vi "SupplySecurityWithoutP2X.vi"(8 "error in (no error)":errorcluster, 11 "DataFlowIN":T2) -> (0 "error out":errorcluster, 3 "DataFlowOUT":T2)   [LabVIEW 2019]
doc: "Subpanel Plugin VI that displays a random value, multiplied by a user-specified value, in a waveform chart."
uses:
  classes/DataCollector.lvclass
  classes/DataHandler.lvclass
panel:
  in  "Abfragegeschwindigkeit DB [ms]":i32=100
  out "Unload Limit":dbl
  out "Load Limit":dbl
  out "Bin-No.":u32
  out "Car enable Signal 2":bool
  out "Distance":bool
  out "E-Car":i32
  out "Car enable":bool
  out "Daytime":i32
  out "buffer":bool
  out "error out 2":errorcluster
  in  "Stopp":bool
  out "Car enable Signal":bool
  in  "Controlling":T1={"Prioritization"=0, "Operating Mode"="", "Release Time "={"Start"=0.0, "Stop"=0.0}, "Activity"=TRUE, " Limitation"={"CPC Power"=0.0, "Unload Power"=0.0, "Load Power"=0.0}}
  in  "Field Elements":i32(listbox)
  out "Control-Matrix-Overview":i32(listbox)=-1
  # "Zone 1 = Bin 1"
  # "Zone 2 = Bin 2"
  # "Zone 3 = Bin 4"
  # "DataCollector.lvclass:SelectValueDC.vi:Step on \"SELECT COUNT(*) FROM ThSorage\"\n\nSQLITE_BUSY(5): database is locked\n\nComplete Call Chain:\nDataCollector.lvclass:SelectValueDC.vi\nForecastNightDay.vi\nForecastSummerWinter.vi\nPrimaryEnergyMinimizationWithoutP2X.vi"
  # "DataCollector.lvclass:SelectValueDC.vi:Step on \"SELECT COUNT(*) FROM 'ElSorage_eCar'\"\n\nSQLITE_BUSY(5): database is locked\n\nComplete Call Chain:\nDataCollector.lvclass:SelectValueDC.vi\nPrimaryEnergyMinimizationWithoutP2X.vi"
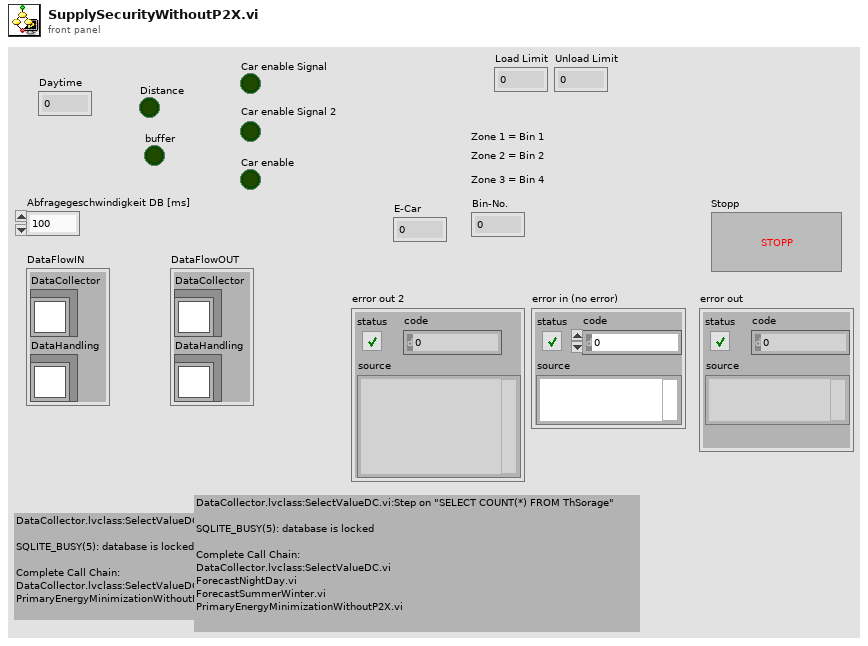
[diagram p1: front panel]
types:
  T1 = cluster{"Prioritization":i8, "Operating Mode":string, "Release Time ":cluster{"Start":dbl, "Stop":dbl}, "Activity":bool, " Limitation":cluster{"CPC Power":dbl, "Unload Power":dbl, "Load Power":dbl}}
  T2 = cluster{"DataCollector":refnum<class "DataCollector.lvclass">, "DataHandling":refnum<class "DataHandler.lvclass">}
  T3 = cluster{"Zone 1":cluster{"TOP_enable_Z1":dbl, "LOW_enable_Z1":dbl, "TOP_disable_Z1":dbl, "LOW_disable_Z1":dbl, "TOP_enable_crit__Z1":dbl, "LOW_enable_crit_Z1":dbl}, "Zone 2":cluster{"TOP_enable_Z2":dbl, "LOW_enable_Z2":dbl, "TOP_disable_Z2":dbl, "LOW_disable_Z2":dbl, "TOP_enable_crit__Z2":dbl, "LOW_enable_crit_Z2":dbl}, "Zone 3":cluster{"TOP_enable_Z3":dbl, "LOW_enable_Z3":dbl, "TOP_disable_Z3":dbl, "LOW_disable_Z3":dbl, "TOP_enable_crit__Z3":dbl, "LOW_enable_crit_Z3":dbl}}
  T4 = cluster{"Activity (on / off)":i64, "Prioritization":i64, "CPC Power Limit":dbl, "Unload Power Limit":dbl, "Load Power Limit":dbl, "Release Time":string, "Operating Mode":string}
  T5 = cluster{"DataCollector out":refnum<class "DataCollector.lvclass">, "DataHandler out":refnum<class "DataHandler.lvclass">}
  T6 = cluster{"TOP_enable_Z1":dbl, "LOW_enable_Z1":dbl, "TOP_disable_Z1":dbl, "LOW_disable_Z1":dbl, "TOP_enable_crit__Z1":dbl, "LOW_enable_crit_Z1":dbl}
  T7 = cluster{"TOP_enable_Z2":dbl, "LOW_enable_Z2":dbl, "TOP_disable_Z2":dbl, "LOW_disable_Z2":dbl, "TOP_enable_crit__Z2":dbl, "LOW_enable_crit_Z2":dbl}
  T8 = cluster{"TOP_enable_Z3":dbl, "LOW_enable_Z3":dbl, "TOP_disable_Z3":dbl, "LOW_disable_Z3":dbl, "TOP_enable_crit__Z3":dbl, "LOW_enable_crit_Z3":dbl}
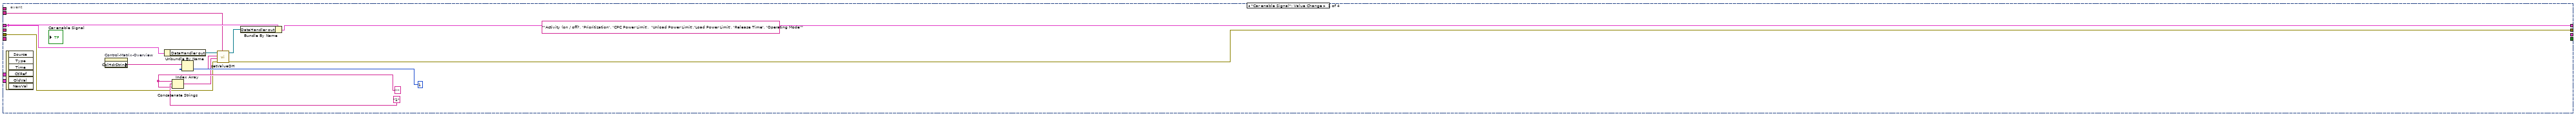
[diagram p2: hidden frame]
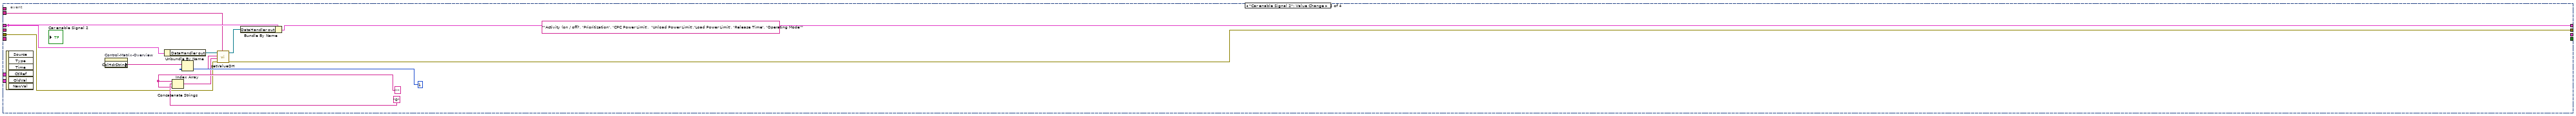
[diagram p3: hidden frame]
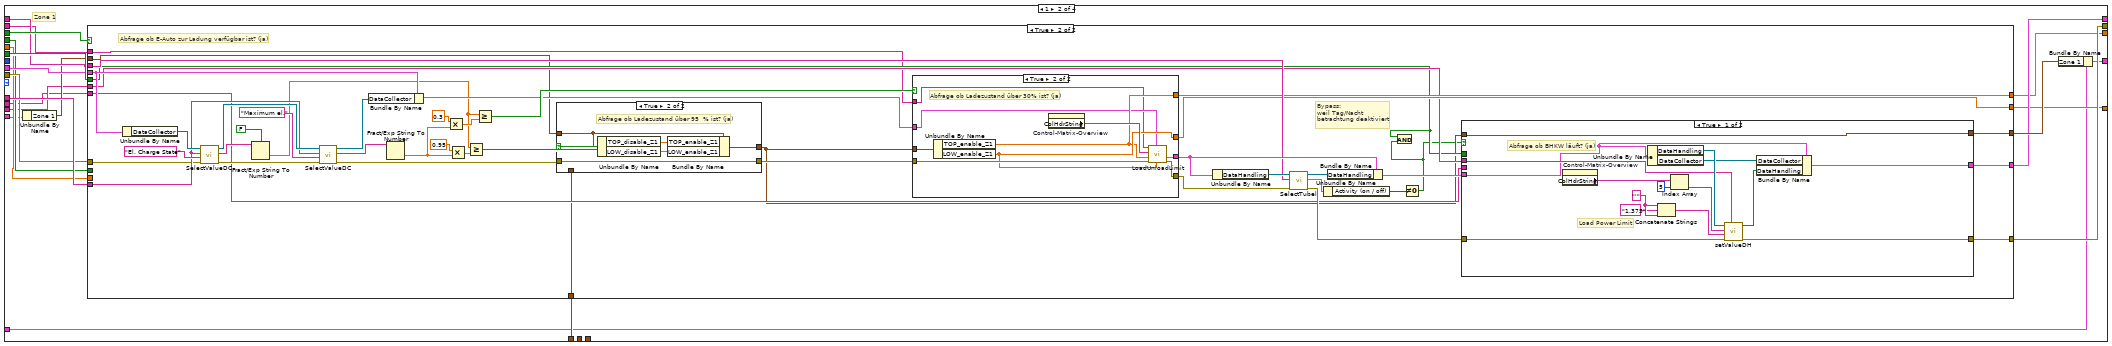
[diagram p5: hidden frame]
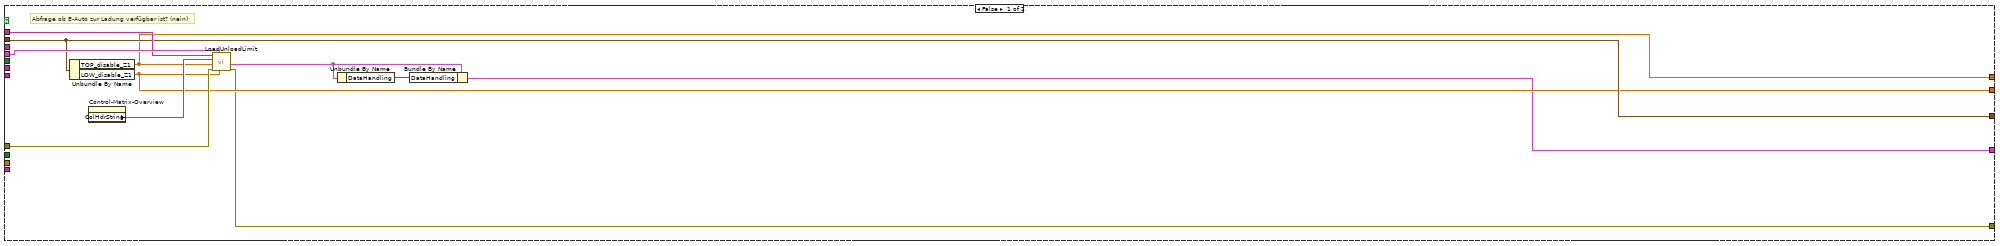
[diagram p6: hidden frame]
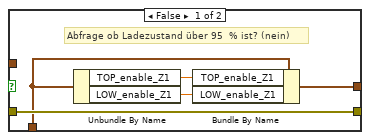
[diagram p7: hidden frame]
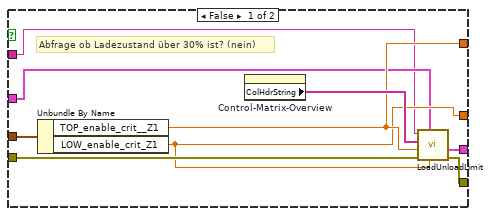
[diagram p8: hidden frame]
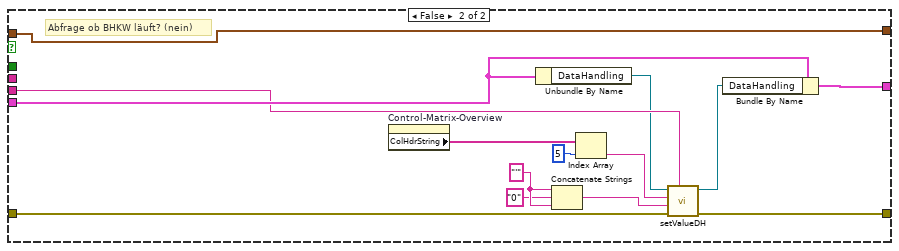
[diagram p9: hidden frame]
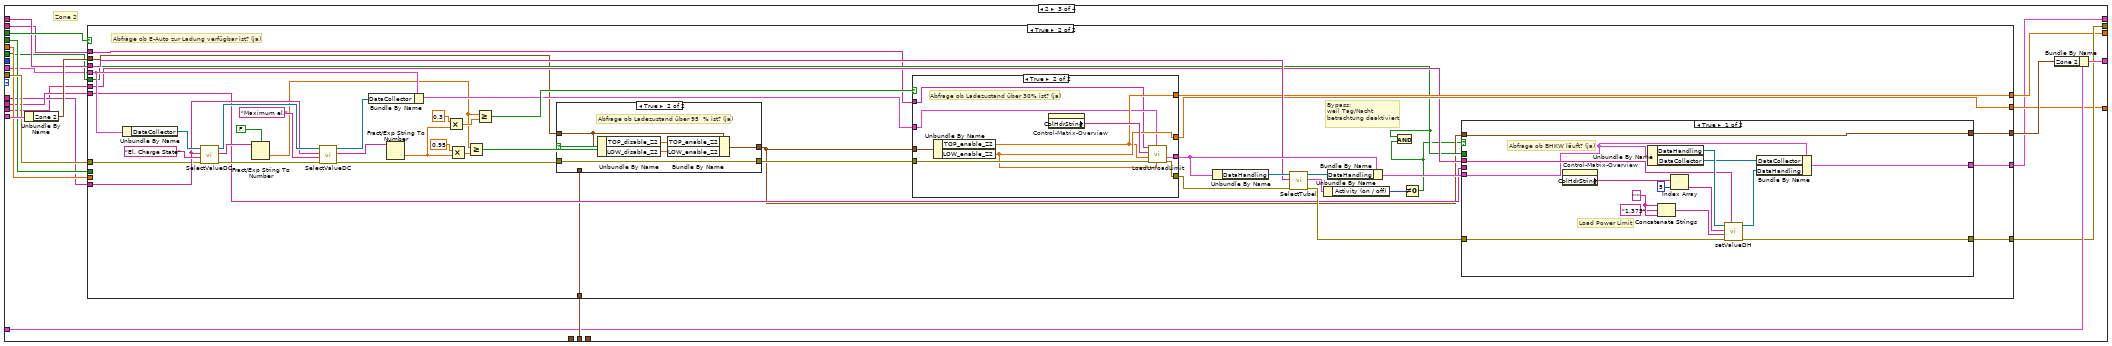
[diagram p10: hidden frame]
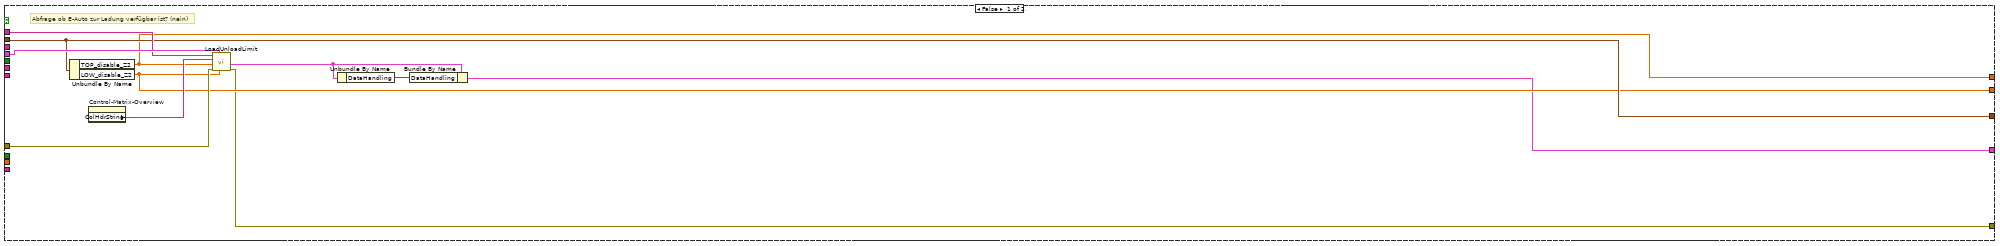
[diagram p11: hidden frame]
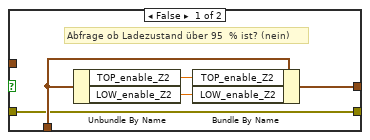
[diagram p12: hidden frame]
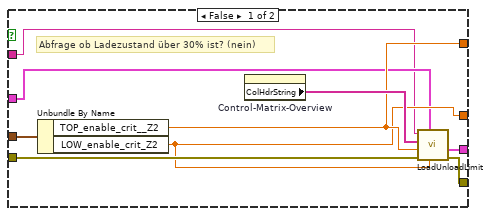
[diagram p13: hidden frame]
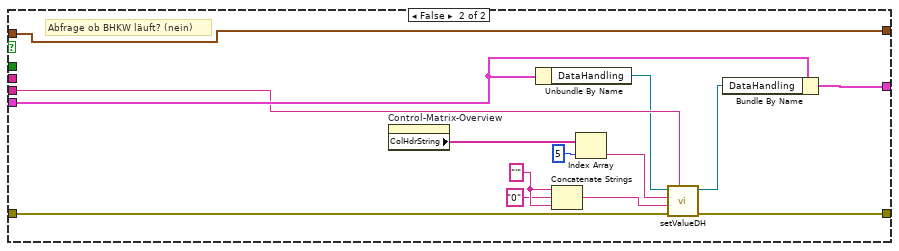
[diagram p14: hidden frame]
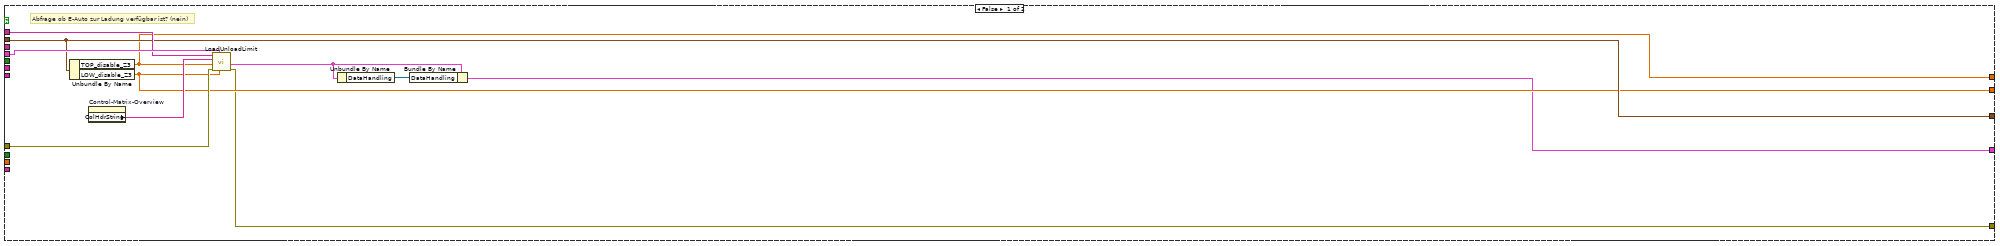
[diagram p15: hidden frame]
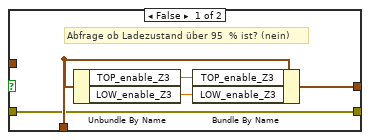
[diagram p16: hidden frame]
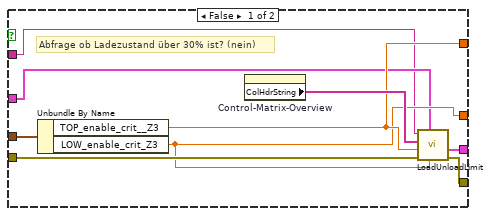
[diagram p17: hidden frame]
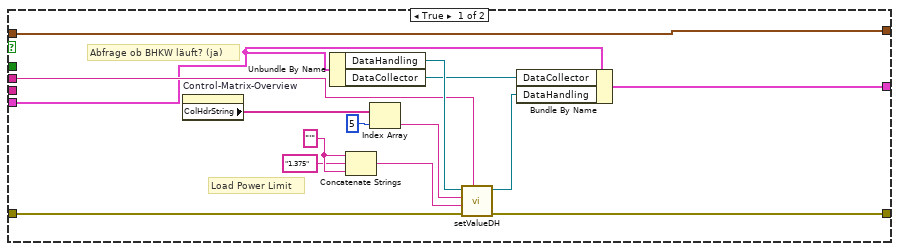
[diagram p18: hidden frame]
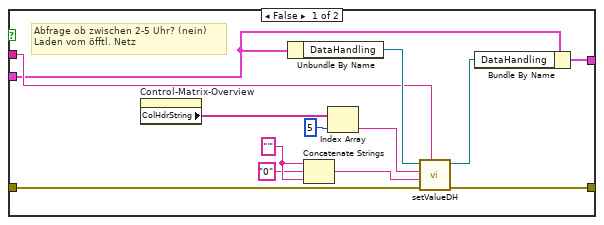
[diagram p19: hidden frame]
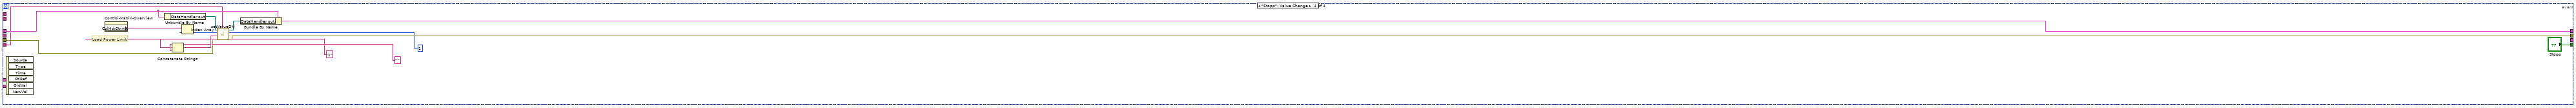
[diagram p20: hidden frame]
diagram:
  w5 = T3 {"Zone 1"={"TOP_enable_Z1"=55.0, "LOW_enable_Z1"=40.0, "TOP_disable_Z1"=50.0, "LOW_disable_Z1"=30.0, "TOP_enable_crit__Z1"=55.0, "LOW_enable_crit_Z1"=50.0}, "Zone 2"={"TOP_enable_Z2"=45.0, "LOW_enable_Z2"=40.0, "TOP_disable_Z2"=40.0, "LOW_disable_Z2"=30.0, "TOP_enable_crit__Z2"=50.0, "LOW_enable_crit_Z2"=45.0}, "Zone 3"={"TOP_enable_Z3"=40.0, "LOW_enable_Z3"=35.0, "TOP_disable_Z3"=35.0, "LOW_disable_Z3"=30.0, "TOP_enable_crit__Z3"=40.0, "LOW_enable_crit_Z3"=37.0}}
  w11 = TRUE
  (unwired) "'Daytime', 'Day of Year', 'El. Energy In',  'El. Energy Out', 'Th. Energy In',  'Th. Energy Out', 'Ch. Energy In',  'Ch. Energy Out',  'Maximum el.', 'Minimal el.', 'Maximum th.', 'Minimal th.',  'Maximum ch.', 'Minimal ch.', 'El. Capacity',  'Th. Capacity', 'Ch. Capacity', 'El. Charge State', 'Th. Charge State',  'Ch. Charge State', 'Activity (on / off)', 'Prioritization', 'El. Power Limitation',  'Th. Power Limitation', 'Ch. Power Limitation', 'Release Time', 'Operating Mode', 'e-Car Load Enable', 'e-Car Mileage  [km]'" ("string")
  w6 = "'CHP'" ("TableName")
  # "SQLite.lvlib:Connection.lvclass:Prepare (pointers).vi\nMAIN db name-->\"C:\\Users\\a_asfe0001\\Desktop\\CHPMobilityEnergySystem\\datebases\\e-car-management_controlling2.db\"\n\nSQLITE_ERROR(1): near \"618182\": syntax error\n\nComplete Call Chain:\nSQLite.lvlib:Connection.lvclass:Prepare (pointers).vi\nSQLite.lvlib:Connection.lvclass:Execute SQL (No results).vi:3980001\nDataHandler.lvclass:setValueDH.vi\nPrimaryEnergyMinimizationWithoutP2X.vi\n\nSQL: \"UPDATE ThSorage SET 'Load Power Limit' = 224,618182;\""
  n1 = case shown="True" w11 {
    tunnel: [w16 w34] -> w4
    tunnel: "error in (no error)" -> [w21 w33]
    tunnel: [w20 w27] -> w9
    tunnel: w6 -> [w19 w25]
    tunnel: [w17 w30] -> _
    frame False {
      n2 = Unbundle By Name("DataFlowIN") -> ("DataHandling"=w23:refnum<class "DataHandler.lvclass">)
      n3 = call-dynamic "SelectTubel.vi"("error in (no error)"=w21, "Unique Object Identifier"=w19, "DataHandler in"=w23) -> ("error out"=w20:errorcluster, "Control Parameter"=w24:T4, "DataHandler out"=w18:refnum<class "DataHandler.lvclass">)  [unwired: 5 in, 1 out]
      n4 = Unbundle By Name(w24) -> ("Activity (on / off)"=w17:i64)
      n5 = Bundle By Name(cluster="DataFlowIN", "DataHandling"=w18) -> (w16:T2)
    }
    frame True {
      w36 = refnum<class "DataHandler.lvclass"> refnum  # DataHandler.lvclass
      w41 = refnum<class "DataCollector.lvclass"> refnum  # DataCollector.lvclass
      n6 = call <vilib>:"Application Directory.vi"() -> ("Application Directory"=w44:path)
      n7 = Build Path(base path=w44, name or relative path="datebases\\e-car-management_monitoring_M12_SLP_gas_20000kWh_15min_500ms.db" ("Name oder relativer Pfad")) -> (appended path=w40:path)
      n8 = call <vilib>:"Application Directory.vi"() -> ("Application Directory"=w38:path)
      n9 = Build Path(base path=w38, name or relative path="datebases/e-car-management_controlling2.db" ("Name oder relativer Pfad")) -> (appended path=w35:path)
      n10 = call-dynamic "OpenCollector.vi"("error in (no error)"=w33, "Ram?"=FALSE, "path to db monitoring"=w40, "DataCollector in"=w41) -> ("error out"=w32:errorcluster, "DataCollector out"=w39:refnum<class "DataCollector.lvclass">)  [unwired: 5 in, 1 out]
      n11 = call-dynamic "OpenHandler.vi"("error in (no error)"=w32, "path to db monitoring"=w35, "DataHandling in"=w36) -> ("error out"=w26:errorcluster, "DataHandling out"=w28:refnum<class "DataHandler.lvclass">)  [unwired: 7 in]
      n12 = call-dynamic "SelectTubel.vi"("error in (no error)"=w26, "Unique Object Identifier"=w25, "DataHandler in"=w28) -> ("error out"=w27:errorcluster, "Control Parameter"=w31:T4, "DataHandler out"=w29:refnum<class "DataHandler.lvclass">)  [unwired: 5 in, 1 out]
      n13 = Unbundle By Name(w31) -> ("Activity (on / off)"=w30:i64)
      n14 = Bundle("DataCollector out"=w39, "DataHandler out"=w29) -> (w34:T5)  [unwired: 1 in]
    }
  }
  n15 = disable-structure shown="Aktiviert" {
    frame Disabled {
      n16 = property on="Eigenschaftsknoten" class="MehrSpaltFeld (strikt)"() -> ("ColHdrString"=w59:string[])  [unwired: 2 in, 2 out]
      n17 = Index Array(array=w59, index=2) -> (element=w57:string)
      n18 = Number To Decimal String(number=9 ("Zahl")) -> (decimal integer string=w60:string)  [unwired: 1 in]
      n19 = call "RestOperatingHoursEl.vi"() -> ("Fehler (Ausgang)"=w47:errorcluster, "DataFlowIN (Ausgang)"=w48:T2, "DataFlowIN (Eingang)"=w49:T2, "TableName"=w46:string)  [unwired: 7 in, 1 out]
      n20 = call-dynamic "setValueDH.vi"("error in (no error)"=w50, "Value"=w60, "ItemName"=w57, "DataHandler in"=w53) -> ("error out"=w55:errorcluster, "DataHandler out"=w52:refnum<class "DataHandler.lvclass">, "TableName"=w51:string)  [unwired: 5 in]
      n21 = call "RestOperatingHours.vi"("Fehler (Eingang, kein Fehler)"=w47, "DataFlowIN (Eingang)"=w48, "TableName"=w51) -> ("Fehler (Ausgang)"=w50:errorcluster, "DataFlowIN (Ausgang)"=w45:T2)  [unwired: 6 in, 1 out]
      n22 = Unbundle By Name(w45) -> ("DataHandling"=w53:refnum<class "DataHandler.lvclass">)
      n23 = Bundle By Name(cluster=w45, "DataHandling"=w52) -> (w54:T2)
    }
    frame Enabled {
    }
  }
  n24 = Unbundle By Name(w5) -> ("Zone 1"=w1:T6, "Zone 2"=w2:T7, "Zone 3"=w3:T8)
  n25 = while {
    tunnel: "ThSorage" ("TableName") -> [w77]
    tunnel: w6 -> [w76]
    tunnel: "'ElSorage_eCar'" ("TableName") -> [w64]
    tunnel: "'Consumer_EF'" ("TableName") -> [w75]
    shift-right: [w67] -> w8
    shift-left: w9 -> [w74]
    shift-right: [w72] -> w12
    shift-left: w4 -> [w71]
    shift-right: [w65] -> _
    shift-left: w5 -> [w66]
    tunnel: w3 -> [w63]
    tunnel: w2 -> [w62]
    tunnel: w1 -> [w61]
    stop <- w68 stop-if-true
    n26 = event shown="[2] Timeout" {
      selector: _ -> [_ _ _ _]
      dyn-events: _ -> [_ _ _ _]
      timeout: "Abfragegeschwindigkeit DB [ms]" -> [_ _ _ _]
      tunnel: w77 -> [_ _ w123 _]
      tunnel: [w90 w103 w110 w578] -> w67
      tunnel: w76 -> [w78 w91 w118 _]
      tunnel: w64 -> [_ _ w108 w575]
      tunnel: w75 -> [_ _ _ _]
      tunnel: w71 -> [w81 w94 w111 w577]
      tunnel: w74 -> [w80 w93 w138 w579]
      tunnel: [w89 w102 w148 w576] -> w72
      tunnel: [_ _ _ "Stopp"] -> w70
      tunnel: w66 -> [_ _ w114 _]
      tunnel: w66 -> [_ _ w113 _]
      tunnel: [_ _ w112 _] -> w65
      tunnel: w63 -> [_ _ w107 _]
      tunnel: w62 -> [_ _ w105 _]
      tunnel: w61 -> [_ _ w104 _]
      event "Car enable Signal": Value Change {
        w84 = "'" ("String")
        (unwired) "'Activity (on / off)', 'Prioritization', 'CPC Power Limit',  'Unload Power Limit','Load Power Limit', 'Release Time', 'Operating Mode'" ("string")
        n27 = event-data() -> ()  [unwired: 1 in, 6 out]
        n28 = property on="Control-Matrix-Overview" class="MehrSpaltFeld (strikt)"() -> ("ColHdrString"=w85:string[])  [unwired: 2 in, 2 out]
        n29 = Unbundle By Name(w81) -> ("DataHandler out"=w79:refnum<class "DataHandler.lvclass">)
        n30 = Concatenate Strings(w84, "1" ("String"), w84) -> (w83:string)
        n31 = Index Array(array=w85, index=1) -> (element=w87:string)
        n32 = call-dynamic "setValueDH.vi"("TableName"=w78, "error in (no error)"=w80, "Value"=w83, "ItemName"=w87, "DataHandler in"=w79) -> ("error out"=w90:errorcluster, "DataHandler out"=w86:refnum<class "DataHandler.lvclass">)  [unwired: 5 in]
        n33 = Bundle By Name(cluster=w81, "DataHandler out"=w86) -> (w89:T5)
      }
      event "Car enable Signal 2": Value Change {
        w97 = "'" ("String")
        (unwired) "'Activity (on / off)', 'Prioritization', 'CPC Power Limit',  'Unload Power Limit','Load Power Limit', 'Release Time', 'Operating Mode'" ("string")
        n34 = event-data() -> ()  [unwired: 1 in, 6 out]
        n35 = property on="Control-Matrix-Overview" class="MehrSpaltFeld (strikt)"() -> ("ColHdrString"=w98:string[])  [unwired: 2 in, 2 out]
        n36 = Unbundle By Name(w94) -> ("DataHandler out"=w92:refnum<class "DataHandler.lvclass">)
        n37 = Concatenate Strings(w97, "0" ("String"), w97) -> (w96:string)
        n38 = Index Array(array=w98, index=1) -> (element=w100:string)
        n39 = call-dynamic "setValueDH.vi"("TableName"=w91, "error in (no error)"=w93, "Value"=w96, "ItemName"=w100, "DataHandler in"=w92) -> ("error out"=w103:errorcluster, "DataHandler out"=w99:refnum<class "DataHandler.lvclass">)  [unwired: 5 in]
        n40 = Bundle By Name(cluster=w94, "DataHandler out"=w99) -> (w102:T5)
      }
      event Timeout {
        # "th"
        n41 = event-data() -> ()  [unwired: 1 in, 3 out]
        n42 = Unbundle By Name(w111) -> ("DataCollector out"=w144:refnum<class "DataCollector.lvclass">, "DataHandler out"=w140:refnum<class "DataHandler.lvclass">)
        n43 = call-dynamic "getControlMatrixDH.vi"("error in (no error)"=w138, "DataHandler in"=w140) -> ("error out"=w137:errorcluster, "List of ColHads"=w141:string[], "ControlParameterArrayMatrix"=w143:string[][], "DataHandler out"=w139:refnum<class "DataHandler.lvclass">, "Field Elements"=w142:string[])  [unwired: 5 in]
        n44 = property on="Field Elements" class="Listenfeld (strikt)"("Item Names"=w142) -> ()  [unwired: 2 in, 2 out]
        n45 = property on="Control-Matrix-Overview" class="MehrSpaltFeld (strikt)"("ItemNames"=w143) -> ()  [unwired: 2 in, 2 out]
        n46 = property on="Control-Matrix-Overview" class="MehrSpaltFeld (strikt)"("ColHdrString"=w141) -> ()  [unwired: 2 in, 2 out]
        n47 = call-dynamic "SelectValueDC.vi"("error in (no error)"=w137, "Table Row Name"="e-Car Load Enable", "Unique Object Identifier"=w108, "DataCollector in"=w144) -> ("error out"=w134:errorcluster, "Value"=w145:string, "DataCollector out"=w135:refnum<class "DataCollector.lvclass">)  [unwired: 5 in]
        n48 = call-dynamic "SelectValueDC.vi"("error in (no error)"=w134, "Table Row Name"="e-Car Mileage  [km]", "Unique Object Identifier"=w108, "DataCollector in"=w135) -> ("error out"=w126:errorcluster, "Value"=w133:string, "DataCollector out"=w128:refnum<class "DataCollector.lvclass">)  [unwired: 5 in]
        n49 = Decimal String To Number(string=w145) -> (number=w146:i32)  [unwired: 2 in, 1 out]
        "E-Car" <- w146
        n50 = Decimal String To Number(string=w133) -> (number=w132:i32)  [unwired: 2 in, 1 out]
        n51 = call-dynamic "SelectValueDC.vi"("error in (no error)"=w126, "Table Row Name"="Th. Charge State", "Unique Object Identifier"=w123, "DataCollector in"=w128) -> ("error out"=w122:errorcluster, "Value"=w106:string, "DataCollector out"=w127:refnum<class "DataCollector.lvclass">)  [unwired: 5 in]
        n52 = Bundle By Name(cluster=w111, "DataCollector out"=w127, "DataHandler out"=w139) -> (w121:T5)
        n53 = Fract/Exp String To Number(string=w106) -> (number=w129:dbl)  [unwired: 3 in, 1 out]
        n54 = Not Equal To 0?(x=w146) -> (x != 0?=w136:bool)
        "Car enable" <- w136
        n55 = Not Equal To 0?(x=w132) -> (x != 0?=w109:bool)
        "Distance" <- w109
        n56 = call "ForecastSummerWinter.vi"("Fehler (Eingang, kein Fehler)"=w122, "DataFlowIN (Eingang)"=w121, "TableName"=w123) -> ("Fehler (Ausgang)"=w124:errorcluster, "DataFlowIN (Ausgang)"=w125:T2, "Daytime"=w120:i32, "Bin-No."=w119:u32, "Night(22-6)?"=w115:bool)  [unwired: 1 in, 3 out]
        "Daytime" <- w120
        "Bin-No." <- w119
        n57 = case shown="4" w119 {
          tunnel: [w151 w157 w286 w428] -> w148
          tunnel: w136 -> [_ w172 w306 w437]
          tunnel: w108 -> [_ w161 w295 w431]
          tunnel: w109 -> [_ w165 w301 w436]
          tunnel: w129 -> [_ w164 w300 w435]
          tunnel: w125 -> [w151 w167 w298 w430]
          tunnel: w124 -> [w150 w166 w303 w438]
          tunnel: w123 -> [_ w168 w294 w433]
          tunnel: w120 -> [_ _ _ _]
          tunnel: w115 -> [_ w171 w299 w429]
          tunnel: w118 -> [_ w169 w302 w434]
          tunnel: [_ w154 w287 w420] -> w117
          tunnel: [_ w155 w288 w427] -> w116
          tunnel: w108 -> [_ w160 w297 w432]
          tunnel: w114 -> [_ w163 w305 w440]
          tunnel: w113 -> [w149 w152 w290 w425]
          tunnel: [w149 w153 w292 w424] -> w112
          tunnel: [w150 w156 w289 w421] -> w110
          tunnel: w108 -> [_ w170 w296 w423]
          tunnel: w107 -> [_ _ _ w422]
          tunnel: w105 -> [_ _ w291 _]
          tunnel: w104 -> [_ w159 _ _]
          frame 0, Default {
          }
          frame 1 {
            # "Zone 1"
            n58 = Unbundle By Name(w163) -> ("Zone 1"=w162:T6)
            n59 = case shown="True" w172 {
              tunnel: [w174 w227] -> w157
              tunnel: [w173 w228] -> w156
              tunnel: w161 -> [_ w197]
              tunnel: w166 -> [w182 w204]
              tunnel: w167 -> [w181 w203]
              tunnel: w168 -> [w179 w186]
              tunnel: w171 -> [_ w196]
              tunnel: w169 -> [_ w206]
              tunnel: [w176 w202] -> w155
              tunnel: w160 -> [_ w198]
              tunnel: w162 -> [w177 w188]
              tunnel: [w177 w226] -> w158
              tunnel: w170 -> [_ w205]
              tunnel: w165 -> [_ _]
              tunnel: w164 -> [_ _]
              tunnel: w159 -> [_ w184]
              tunnel: [w175 w201] -> w154
              frame False {
                # "Abfrage ob E-Auto zur Ladung verfügbar ist? (nein)"
                n60 = Unbundle By Name(w177) -> ("TOP_disable_Z1"=w175:dbl, "LOW_disable_Z1"=w176:dbl)
                n61 = property on="Control-Matrix-Overview" class="MehrSpaltFeld (strikt)"() -> ("ColHdrString"=w178:string[])  [unwired: 2 in, 2 out]
                n62 = call "LoadUnloadLimit.vi"("Unload Limit"=w176, "DataFlowIN (Eingang)"=w181, "Fehler (Eingang, kein Fehler)"=w182, "Load Limit"=w175, "ColHdrString"=w178, "TableName"=w179) -> ("Fehler (Ausgang)"=w173:errorcluster, "DataFlowIN (Ausgang)"=w180:T2)  [unwired: 2 in, 2 out]
                n63 = Unbundle By Name(w180) -> ("DataHandling"=w183:refnum<class "DataHandler.lvclass">)
                n64 = Bundle By Name(cluster=w180, "DataHandling"=w183) -> (w174:T2)
              }
              frame True {
                # "Bypass:\nweil Tag/Nacht \nbetrachtung deaktiviert"
                # "Abfrage ob E-Auto zur Ladung verfügbar ist? (ja)"
                n65 = Unbundle By Name(w203) -> ("DataCollector"=w216:refnum<class "DataCollector.lvclass">)
                n66 = call-dynamic "SelectValueDC.vi"("error in (no error)"=w204, "Table Row Name"="El. Charge State", "Unique Object Identifier"=w205, "DataCollector in"=w216) -> ("error out"=w212:errorcluster, "Value"=w213:string, "DataCollector out"=w215:refnum<class "DataCollector.lvclass">)  [unwired: 5 in]
                n67 = Fract/Exp String To Number(use system decimal point (T)=FALSE ("Systemdezimalzeichen verwenden (T)"), string=w213) -> (number=w192:dbl)  [unwired: 2 in, 1 out]
                n68 = call-dynamic "SelectValueDC.vi"("error in (no error)"=w212, "Table Row Name"="Maximum el.", "Unique Object Identifier"=w205, "DataCollector in"=w215) -> ("error out"=w190:errorcluster, "Value"=w211:string, "DataCollector out"=w214:refnum<class "DataCollector.lvclass">)  [unwired: 5 in]
                n69 = Bundle By Name(cluster=w203, "DataCollector"=w214) -> (w217:T2)
                n70 = Fract/Exp String To Number(string=w211) -> (number=w193:dbl)  [unwired: 3 in, 1 out]
                n71 = Multiply(x=0.3 ("x*y"), y=w193) -> (x*y=w219:dbl)
                n72 = Multiply(x=0.95 ("x*y"), y=w193) -> (x*y=w194:dbl)
                n73 = Greater Or Equal?(x=w192, y=w194) -> (x >= y?=w191:bool)
                n74 = Greater Or Equal?(x=w192, y=w219) -> (x >= y?=w218:bool)
                n75 = case shown="True" w191 {
                  tunnel: w188 -> [_ w234]
                  tunnel: [w231 w235] -> w187
                  tunnel: [w230 w238] -> w189
                  tunnel: w190 -> [w230 w238]
                  tunnel: w184 -> [w229 _]
                  frame False {
                    # "Abfrage ob Ladezustand über 95  % ist? (nein)"
                    n76 = Unbundle By Name(w229) -> ("TOP_enable_Z1"=w232:dbl, "LOW_enable_Z1"=w233:dbl)
                    n77 = Bundle By Name(cluster=w229, "TOP_enable_Z1"=w232, "LOW_enable_Z1"=w233) -> (w231:T6)
                  }
                  frame True {
                    # "Abfrage ob Ladezustand über 95  % ist? (ja)"
                    n78 = Unbundle By Name(w234) -> ("TOP_disable_Z1"=w236:dbl, "LOW_disable_Z1"=w237:dbl)
                    n79 = Bundle By Name(cluster=w234, "TOP_enable_Z1"=w236, "LOW_enable_Z1"=w237) -> (w235:T6)
                  }
                }
                n80 = case shown="True" w218 {
                  tunnel: [w243 w251] -> w221
                  tunnel: w217 -> [w240 w250]
                  tunnel: w189 -> [w246 w255]
                  tunnel: [w242 w252] -> w220
                  tunnel: [w245 w253] -> w201
                  tunnel: [w244 w254] -> w202
                  tunnel: w186 -> [w239 w249]
                  tunnel: w187 -> [w241 w248]
                  frame False {
                    # "Abfrage ob Ladezustand über 30% ist? (nein)"
                    n81 = Unbundle By Name(w241) -> ("TOP_enable_crit__Z1"=w245:dbl, "LOW_enable_crit_Z1"=w244:dbl)
                    n82 = property on="Control-Matrix-Overview" class="MehrSpaltFeld (strikt)"() -> ("ColHdrString"=w247:string[])  [unwired: 2 in, 2 out]
                    n83 = call "LoadUnloadLimit.vi"("Unload Limit"=w244, "DataFlowIN (Eingang)"=w240, "Fehler (Eingang, kein Fehler)"=w246, "Load Limit"=w245, "ColHdrString"=w247, "TableName"=w239) -> ("Fehler (Ausgang)"=w242:errorcluster, "DataFlowIN (Ausgang)"=w243:T2)  [unwired: 2 in, 2 out]
                  }
                  frame True {
                    # "Abfrage ob Ladezustand über 30% ist? (ja)"
                    n84 = Unbundle By Name(w248) -> ("TOP_enable_Z1"=w253:dbl, "LOW_enable_Z1"=w254:dbl)
                    n85 = property on="Control-Matrix-Overview" class="MehrSpaltFeld (strikt)"() -> ("ColHdrString"=w256:string[])  [unwired: 2 in, 2 out]
                    n86 = call "LoadUnloadLimit.vi"("Unload Limit"=w254, "DataFlowIN (Eingang)"=w250, "Fehler (Eingang, kein Fehler)"=w255, "Load Limit"=w253, "ColHdrString"=w256, "TableName"=w249) -> ("Fehler (Ausgang)"=w252:errorcluster, "DataFlowIN (Ausgang)"=w251:T2)  [unwired: 2 in, 2 out]
                  }
                }
                n87 = Unbundle By Name(w221) -> ("DataHandling"=w225:refnum<class "DataHandler.lvclass">)
                n88 = call-dynamic "SelectTubel.vi"("error in (no error)"=w220, "Unique Object Identifier"=w206, "DataHandler in"=w225) -> ("error out"=w200:errorcluster, "Control Parameter"=w223:T4, "DataHandler out"=w224:refnum<class "DataHandler.lvclass">)  [unwired: 5 in, 1 out]
                n89 = Unbundle By Name(w223) -> ("Activity (on / off)"=w222:i64)
                n90 = Bundle By Name(cluster=w221, "DataHandling"=w224) -> (w199:T2)
                n91 = Not Equal To 0?(x=w222) -> (x != 0?=w185:bool)
                n92 = And(x=w196, y=w185) -> ()  [unwired: 1 out]
                n93 = case shown="True" w185 {
                  tunnel: [w261 w285] -> w228
                  tunnel: [w257 w284] -> w227
                  tunnel: w197 -> [w267 _]
                  tunnel: w200 -> [w265 w283]
                  tunnel: w199 -> [w258 w282]
                  tunnel: w198 -> [_ w281]
                  tunnel: w187 -> [w262 w280]
                  tunnel: [w262 w280] -> w226
                  tunnel: w196 -> [_ _]
                  frame True {
                    w266 = "'" ("String")
                    # "Abfrage ob BHKW läuft? (ja)"
                    # "Load Power Limit"
                    n94 = property on="Control-Matrix-Overview" class="MehrSpaltFeld (strikt)"() -> ("ColHdrString"=w263:string[])  [unwired: 2 in, 2 out]
                    n95 = Unbundle By Name(w258) -> ("DataHandling"=w268:refnum<class "DataHandler.lvclass">, "DataCollector"=w260:refnum<class "DataCollector.lvclass">)
                    n96 = Concatenate Strings(w266, "1.375" ("String"), w266) -> (w269:string)
                    n97 = Index Array(array=w263, index=5) -> (element=w270:string)
                    n98 = call-dynamic "setValueDH.vi"("TableName"=w267, "error in (no error)"=w265, "Value"=w269, "ItemName"=w270, "DataHandler in"=w268) -> ("error out"=w261:errorcluster, "DataHandler out"=w259:refnum<class "DataHandler.lvclass">)  [unwired: 5 in]
                    n99 = Bundle By Name(cluster=w258, "DataCollector"=w260, "DataHandling"=w259) -> (w257:T2)
                  }
                  frame False {
                    w274 = "'" ("String")
                    # "Abfrage ob BHKW läuft? (nein)"
                    n100 = property on="Control-Matrix-Overview" class="MehrSpaltFeld (strikt)"() -> ("ColHdrString"=w272:string[])  [unwired: 2 in, 2 out]
                    n101 = Unbundle By Name(w282) -> ("DataHandling"=w279:refnum<class "DataHandler.lvclass">)
                    n102 = Concatenate Strings(w274, "0" ("String"), w274) -> (w276:string)
                    n103 = Index Array(array=w272, index=5) -> (element=w278:string)
                    n104 = call-dynamic "setValueDH.vi"("TableName"=w281, "error in (no error)"=w283, "Value"=w276, "ItemName"=w278, "DataHandler in"=w279) -> ("error out"=w285:errorcluster, "DataHandler out"=w277:refnum<class "DataHandler.lvclass">)  [unwired: 5 in]
                    n105 = Bundle By Name(cluster=w282, "DataHandling"=w277) -> (w284:T2)
                  }
                }
              }
            }
            n106 = Bundle By Name(cluster=w152, "Zone 1"=w158) -> (w153:T3)
          }
          frame 2 {
            # "Zone 2"
            n107 = Unbundle By Name(w305) -> ("Zone 2"=w304:T7)
            n108 = case shown="True" w306 {
              tunnel: [w308 w361] -> w286
              tunnel: [w307 w362] -> w289
              tunnel: w295 -> [_ w331]
              tunnel: w303 -> [w316 w338]
              tunnel: w298 -> [w315 w337]
              tunnel: w294 -> [w313 w320]
              tunnel: w299 -> [_ w330]
              tunnel: w302 -> [_ w340]
              tunnel: [w309 w335] -> w287
              tunnel: [w310 w336] -> w288
              tunnel: w297 -> [_ w332]
              tunnel: w304 -> [w311 w322]
              tunnel: [w311 w360] -> w293
              tunnel: w296 -> [_ w339]
              tunnel: w301 -> [_ _]
              tunnel: w300 -> [_ _]
              tunnel: w291 -> [_ w318]
              frame False {
                # "Abfrage ob E-Auto zur Ladung verfügbar ist? (nein)"
                n109 = Unbundle By Name(w311) -> ("TOP_disable_Z2"=w309:dbl, "LOW_disable_Z2"=w310:dbl)
                n110 = property on="Control-Matrix-Overview" class="MehrSpaltFeld (strikt)"() -> ("ColHdrString"=w312:string[])  [unwired: 2 in, 2 out]
                n111 = call "LoadUnloadLimit.vi"("Unload Limit"=w310, "DataFlowIN (Eingang)"=w315, "Fehler (Eingang, kein Fehler)"=w316, "Load Limit"=w309, "ColHdrString"=w312, "TableName"=w313) -> ("Fehler (Ausgang)"=w307:errorcluster, "DataFlowIN (Ausgang)"=w314:T2)  [unwired: 2 in, 2 out]
                n112 = Unbundle By Name(w314) -> ("DataHandling"=w317:refnum<class "DataHandler.lvclass">)
                n113 = Bundle By Name(cluster=w314, "DataHandling"=w317) -> (w308:T2)
              }
              frame True {
                # "Bypass:\nweil Tag/Nacht \nbetrachtung deaktiviert"
                # "Abfrage ob E-Auto zur Ladung verfügbar ist? (ja)"
                n114 = Unbundle By Name(w337) -> ("DataCollector"=w350:refnum<class "DataCollector.lvclass">)
                n115 = call-dynamic "SelectValueDC.vi"("error in (no error)"=w338, "Table Row Name"="El. Charge State", "Unique Object Identifier"=w339, "DataCollector in"=w350) -> ("error out"=w346:errorcluster, "Value"=w347:string, "DataCollector out"=w349:refnum<class "DataCollector.lvclass">)  [unwired: 5 in]
                n116 = Fract/Exp String To Number(use system decimal point (T)=FALSE ("Systemdezimalzeichen verwenden (T)"), string=w347) -> (number=w326:dbl)  [unwired: 2 in, 1 out]
                n117 = call-dynamic "SelectValueDC.vi"("error in (no error)"=w346, "Table Row Name"="Maximum el.", "Unique Object Identifier"=w339, "DataCollector in"=w349) -> ("error out"=w324:errorcluster, "Value"=w345:string, "DataCollector out"=w348:refnum<class "DataCollector.lvclass">)  [unwired: 5 in]
                n118 = Bundle By Name(cluster=w337, "DataCollector"=w348) -> (w351:T2)
                n119 = Fract/Exp String To Number(string=w345) -> (number=w327:dbl)  [unwired: 3 in, 1 out]
                n120 = Multiply(x=0.3 ("x*y"), y=w327) -> (x*y=w353:dbl)
                n121 = Multiply(x=0.95 ("x*y"), y=w327) -> (x*y=w328:dbl)
                n122 = Greater Or Equal?(x=w326, y=w328) -> (x >= y?=w325:bool)
                n123 = Greater Or Equal?(x=w326, y=w353) -> (x >= y?=w352:bool)
                n124 = case shown="True" w325 {
                  tunnel: w322 -> [_ w368]
                  tunnel: [w365 w369] -> w321
                  tunnel: w318 -> [w364 _]
                  tunnel: [w363 w372] -> w323
                  tunnel: w324 -> [w363 w372]
                  frame False {
                    # "Abfrage ob Ladezustand über 95  % ist? (nein)"
                    n125 = Unbundle By Name(w364) -> ("TOP_enable_Z2"=w366:dbl, "LOW_enable_Z2"=w367:dbl)
                    n126 = Bundle By Name(cluster=w364, "TOP_enable_Z2"=w366, "LOW_enable_Z2"=w367) -> (w365:T7)
                  }
                  frame True {
                    # "Abfrage ob Ladezustand über 95  % ist? (ja)"
                    n127 = Unbundle By Name(w368) -> ("TOP_disable_Z2"=w370:dbl, "LOW_disable_Z2"=w371:dbl)
                    n128 = Bundle By Name(cluster=w368, "TOP_enable_Z2"=w370, "LOW_enable_Z2"=w371) -> (w369:T7)
                  }
                }
                n129 = case shown="True" w352 {
                  tunnel: [w377 w385] -> w355
                  tunnel: w351 -> [w374 w384]
                  tunnel: w323 -> [w380 w389]
                  tunnel: [w376 w386] -> w354
                  tunnel: [w379 w387] -> w335
                  tunnel: [w378 w388] -> w336
                  tunnel: w320 -> [w373 w383]
                  tunnel: w321 -> [w375 w382]
                  frame False {
                    # "Abfrage ob Ladezustand über 30% ist? (nein)"
                    n130 = Unbundle By Name(w375) -> ("TOP_enable_crit__Z2"=w379:dbl, "LOW_enable_crit_Z2"=w378:dbl)
                    n131 = property on="Control-Matrix-Overview" class="MehrSpaltFeld (strikt)"() -> ("ColHdrString"=w381:string[])  [unwired: 2 in, 2 out]
                    n132 = call "LoadUnloadLimit.vi"("Unload Limit"=w378, "DataFlowIN (Eingang)"=w374, "Fehler (Eingang, kein Fehler)"=w380, "Load Limit"=w379, "ColHdrString"=w381, "TableName"=w373) -> ("Fehler (Ausgang)"=w376:errorcluster, "DataFlowIN (Ausgang)"=w377:T2)  [unwired: 2 in, 2 out]
                  }
                  frame True {
                    # "Abfrage ob Ladezustand über 30% ist? (ja)"
                    n133 = Unbundle By Name(w382) -> ("TOP_enable_Z2"=w387:dbl, "LOW_enable_Z2"=w388:dbl)
                    n134 = property on="Control-Matrix-Overview" class="MehrSpaltFeld (strikt)"() -> ("ColHdrString"=w390:string[])  [unwired: 2 in, 2 out]
                    n135 = call "LoadUnloadLimit.vi"("Unload Limit"=w388, "DataFlowIN (Eingang)"=w384, "Fehler (Eingang, kein Fehler)"=w389, "Load Limit"=w387, "ColHdrString"=w390, "TableName"=w383) -> ("Fehler (Ausgang)"=w386:errorcluster, "DataFlowIN (Ausgang)"=w385:T2)  [unwired: 2 in, 2 out]
                  }
                }
                n136 = Unbundle By Name(w355) -> ("DataHandling"=w359:refnum<class "DataHandler.lvclass">)
                n137 = call-dynamic "SelectTubel.vi"("error in (no error)"=w354, "Unique Object Identifier"=w340, "DataHandler in"=w359) -> ("error out"=w334:errorcluster, "Control Parameter"=w357:T4, "DataHandler out"=w358:refnum<class "DataHandler.lvclass">)  [unwired: 5 in, 1 out]
                n138 = Unbundle By Name(w357) -> ("Activity (on / off)"=w356:i64)
                n139 = Bundle By Name(cluster=w355, "DataHandling"=w358) -> (w333:T2)
                n140 = Not Equal To 0?(x=w356) -> (x != 0?=w319:bool)
                n141 = And(x=w330, y=w319) -> ()  [unwired: 1 out]
                n142 = case shown="True" w319 {
                  tunnel: [w395 w419] -> w362
                  tunnel: [w391 w418] -> w361
                  tunnel: w331 -> [w401 _]
                  tunnel: w334 -> [w399 w417]
                  tunnel: w333 -> [w392 w416]
                  tunnel: w332 -> [_ w415]
                  tunnel: w321 -> [w396 w414]
                  tunnel: [w396 w414] -> w360
                  tunnel: w330 -> [_ _]
                  frame True {
                    w400 = "'" ("String")
                    # "Abfrage ob BHKW läuft? (ja)"
                    # "Load Power Limit"
                    n143 = property on="Control-Matrix-Overview" class="MehrSpaltFeld (strikt)"() -> ("ColHdrString"=w397:string[])  [unwired: 2 in, 2 out]
                    n144 = Unbundle By Name(w392) -> ("DataHandling"=w402:refnum<class "DataHandler.lvclass">, "DataCollector"=w394:refnum<class "DataCollector.lvclass">)
                    n145 = Concatenate Strings(w400, "1.375" ("String"), w400) -> (w403:string)
                    n146 = Index Array(array=w397, index=5) -> (element=w404:string)
                    n147 = call-dynamic "setValueDH.vi"("TableName"=w401, "error in (no error)"=w399, "Value"=w403, "ItemName"=w404, "DataHandler in"=w402) -> ("error out"=w395:errorcluster, "DataHandler out"=w393:refnum<class "DataHandler.lvclass">)  [unwired: 5 in]
                    n148 = Bundle By Name(cluster=w392, "DataCollector"=w394, "DataHandling"=w393) -> (w391:T2)
                  }
                  frame False {
                    w408 = "'" ("String")
                    # "Abfrage ob BHKW läuft? (nein)"
                    n149 = property on="Control-Matrix-Overview" class="MehrSpaltFeld (strikt)"() -> ("ColHdrString"=w406:string[])  [unwired: 2 in, 2 out]
                    n150 = Unbundle By Name(w416) -> ("DataHandling"=w413:refnum<class "DataHandler.lvclass">)
                    n151 = Concatenate Strings(w408, "0" ("String"), w408) -> (w410:string)
                    n152 = Index Array(array=w406, index=5) -> (element=w412:string)
                    n153 = call-dynamic "setValueDH.vi"("TableName"=w415, "error in (no error)"=w417, "Value"=w410, "ItemName"=w412, "DataHandler in"=w413) -> ("error out"=w419:errorcluster, "DataHandler out"=w411:refnum<class "DataHandler.lvclass">)  [unwired: 5 in]
                    n154 = Bundle By Name(cluster=w416, "DataHandling"=w411) -> (w418:T2)
                  }
                }
              }
            }
            n155 = Bundle By Name(cluster=w290, "Zone 2"=w293) -> (w292:T3)
          }
          frame 4 {
            # "Zone 3"
            n156 = Unbundle By Name(w440) -> ("Zone 3"=w439:T8)
            n157 = case shown="True" w437 {
              tunnel: [w442 w495] -> w428
              tunnel: [w441 w496] -> w421
              tunnel: w431 -> [_ w465]
              tunnel: w438 -> [w450 w472]
              tunnel: w430 -> [w449 w471]
              tunnel: w433 -> [w447 w453]
              tunnel: w429 -> [_ w464]
              tunnel: w434 -> [_ w474]
              tunnel: [w443 w469] -> w420
              tunnel: [w444 w470] -> w427
              tunnel: w432 -> [_ w466]
              tunnel: w439 -> [w445 w455]
              tunnel: [w445 w494] -> w426
              tunnel: w436 -> [_ _]
              tunnel: w435 -> [_ _]
              tunnel: w423 -> [_ w473]
              tunnel: w422 -> [_ w458]
              frame False {
                # "Abfrage ob E-Auto zur Ladung verfügbar ist? (nein)"
                n158 = Unbundle By Name(w445) -> ("TOP_disable_Z3"=w443:dbl, "LOW_disable_Z3"=w444:dbl)
                n159 = property on="Control-Matrix-Overview" class="MehrSpaltFeld (strikt)"() -> ("ColHdrString"=w446:string[])  [unwired: 2 in, 2 out]
                n160 = call "LoadUnloadLimit.vi"("Unload Limit"=w444, "DataFlowIN (Eingang)"=w449, "Fehler (Eingang, kein Fehler)"=w450, "Load Limit"=w443, "ColHdrString"=w446, "TableName"=w447) -> ("Fehler (Ausgang)"=w441:errorcluster, "DataFlowIN (Ausgang)"=w448:T2)  [unwired: 2 in, 2 out]
                n161 = Unbundle By Name(w448) -> ("DataHandling"=w451:refnum<class "DataHandler.lvclass">)
                n162 = Bundle By Name(cluster=w448, "DataHandling"=w451) -> (w442:T2)
              }
              frame True {
                # "Bypass:\nweil Tag/Nacht \nbetrachtung deaktiviert"
                # "Abfrage ob E-Auto zur Ladung verfügbar ist? (ja)"
                n163 = Unbundle By Name(w471) -> ("DataCollector"=w484:refnum<class "DataCollector.lvclass">)
                n164 = call-dynamic "SelectValueDC.vi"("error in (no error)"=w472, "Table Row Name"="El. Charge State", "Unique Object Identifier"=w473, "DataCollector in"=w484) -> ("error out"=w480:errorcluster, "Value"=w481:string, "DataCollector out"=w483:refnum<class "DataCollector.lvclass">)  [unwired: 5 in]
                n165 = Fract/Exp String To Number(use system decimal point (T)=FALSE ("Systemdezimalzeichen verwenden (T)"), string=w481) -> (number=w460:dbl)  [unwired: 2 in, 1 out]
                n166 = call-dynamic "SelectValueDC.vi"("error in (no error)"=w480, "Table Row Name"="Maximum el.", "Unique Object Identifier"=w473, "DataCollector in"=w483) -> ("error out"=w457:errorcluster, "Value"=w479:string, "DataCollector out"=w482:refnum<class "DataCollector.lvclass">)  [unwired: 5 in]
                n167 = Bundle By Name(cluster=w471, "DataCollector"=w482) -> (w485:T2)
                n168 = Fract/Exp String To Number(string=w479) -> (number=w461:dbl)  [unwired: 3 in, 1 out]
                n169 = Multiply(x=0.3 ("x*y"), y=w461) -> (x*y=w487:dbl)
                n170 = Multiply(x=0.95 ("x*y"), y=w461) -> (x*y=w462:dbl)
                n171 = Greater Or Equal?(x=w460, y=w462) -> (x >= y?=w459:bool)
                n172 = Greater Or Equal?(x=w460, y=w487) -> (x >= y?=w486:bool)
                n173 = case shown="True" w459 {
                  tunnel: w455 -> [_ w502]
                  tunnel: [w499 w503] -> w454
                  tunnel: w458 -> [w498 _]
                  tunnel: [w497 w506] -> w456
                  tunnel: w457 -> [w497 w506]
                  frame False {
                    # "Abfrage ob Ladezustand über 95  % ist? (nein)"
                    n174 = Unbundle By Name(w498) -> ("TOP_enable_Z3"=w500:dbl, "LOW_enable_Z3"=w501:dbl)
                    n175 = Bundle By Name(cluster=w498, "TOP_enable_Z3"=w500, "LOW_enable_Z3"=w501) -> (w499:T8)
                  }
                  frame True {
                    # "Abfrage ob Ladezustand über 95  % ist? (ja)"
                    n176 = Unbundle By Name(w502) -> ("TOP_disable_Z3"=w504:dbl, "LOW_disable_Z3"=w505:dbl)
                    n177 = Bundle By Name(cluster=w502, "TOP_enable_Z3"=w504, "LOW_enable_Z3"=w505) -> (w503:T8)
                  }
                }
                n178 = case shown="True" w486 {
                  tunnel: [w511 w519] -> w489
                  tunnel: w485 -> [w508 w518]
                  tunnel: w456 -> [w514 w523]
                  tunnel: [w510 w520] -> w488
                  tunnel: [w513 w521] -> w469
                  tunnel: [w512 w522] -> w470
                  tunnel: w453 -> [w507 w517]
                  tunnel: w454 -> [w509 w516]
                  frame False {
                    # "Abfrage ob Ladezustand über 30% ist? (nein)"
                    n179 = Unbundle By Name(w509) -> ("TOP_enable_crit__Z3"=w513:dbl, "LOW_enable_crit_Z3"=w512:dbl)
                    n180 = property on="Control-Matrix-Overview" class="MehrSpaltFeld (strikt)"() -> ("ColHdrString"=w515:string[])  [unwired: 2 in, 2 out]
                    n181 = call "LoadUnloadLimit.vi"("Unload Limit"=w512, "DataFlowIN (Eingang)"=w508, "Fehler (Eingang, kein Fehler)"=w514, "Load Limit"=w513, "ColHdrString"=w515, "TableName"=w507) -> ("Fehler (Ausgang)"=w510:errorcluster, "DataFlowIN (Ausgang)"=w511:T2)  [unwired: 2 in, 2 out]
                  }
                  frame True {
                    # "Abfrage ob Ladezustand über 30% ist? (ja)"
                    n182 = Unbundle By Name(w516) -> ("TOP_enable_Z3"=w521:dbl, "LOW_enable_Z3"=w522:dbl)
                    n183 = property on="Control-Matrix-Overview" class="MehrSpaltFeld (strikt)"() -> ("ColHdrString"=w524:string[])  [unwired: 2 in, 2 out]
                    n184 = call "LoadUnloadLimit.vi"("Unload Limit"=w522, "DataFlowIN (Eingang)"=w518, "Fehler (Eingang, kein Fehler)"=w523, "Load Limit"=w521, "ColHdrString"=w524, "TableName"=w517) -> ("Fehler (Ausgang)"=w520:errorcluster, "DataFlowIN (Ausgang)"=w519:T2)  [unwired: 2 in, 2 out]
                  }
                }
                n185 = Unbundle By Name(w489) -> ("DataHandling"=w493:refnum<class "DataHandler.lvclass">)
                n186 = call-dynamic "SelectTubel.vi"("error in (no error)"=w488, "Unique Object Identifier"=w474, "DataHandler in"=w493) -> ("error out"=w468:errorcluster, "Control Parameter"=w491:T4, "DataHandler out"=w492:refnum<class "DataHandler.lvclass">)  [unwired: 5 in, 1 out]
                n187 = Unbundle By Name(w491) -> ("Activity (on / off)"=w490:i64)
                n188 = Bundle By Name(cluster=w489, "DataHandling"=w492) -> (w467:T2)
                n189 = Not Equal To 0?(x=w490) -> (x != 0?=w452:bool)
                n190 = And(x=w464, y=w452) -> ()  [unwired: 1 out]
                n191 = case shown="False" w452 {
                  tunnel: [w529 w548] -> w496
                  tunnel: [w525 w547] -> w495
                  tunnel: w465 -> [w535 _]
                  tunnel: w468 -> [w533 w546]
                  tunnel: w467 -> [w526 w545]
                  tunnel: w466 -> [_ w544]
                  tunnel: w454 -> [w530 w540]
                  tunnel: [w530 w540] -> w494
                  tunnel: w464 -> [_ w542]
                  frame True {
                    w534 = "'" ("String")
                    # "Abfrage ob BHKW läuft? (ja)"
                    # "Load Power Limit"
                    n192 = property on="Control-Matrix-Overview" class="MehrSpaltFeld (strikt)"() -> ("ColHdrString"=w531:string[])  [unwired: 2 in, 2 out]
                    n193 = Unbundle By Name(w526) -> ("DataHandling"=w536:refnum<class "DataHandler.lvclass">, "DataCollector"=w528:refnum<class "DataCollector.lvclass">)
                    n194 = Concatenate Strings(w534, "1.375" ("String"), w534) -> (w537:string)
                    n195 = Index Array(array=w531, index=5) -> (element=w538:string)
                    n196 = call-dynamic "setValueDH.vi"("TableName"=w535, "error in (no error)"=w533, "Value"=w537, "ItemName"=w538, "DataHandler in"=w536) -> ("error out"=w529:errorcluster, "DataHandler out"=w527:refnum<class "DataHandler.lvclass">)  [unwired: 5 in]
                    n197 = Bundle By Name(cluster=w526, "DataCollector"=w528, "DataHandling"=w527) -> (w525:T2)
                  }
                  frame False {
                    # "Bypass-\nMöglichkeit"
                    # "Abfrage ob BHKW läuft? (nein)"
                    n198 = And(x=w542, y=TRUE) -> (x .and. y?=w543:bool)
                    n199 = case shown="True" w543 {
                      tunnel: w545 -> [w553 w565]
                      tunnel: w546 -> [w552 w564]
                      tunnel: [w551 w563] -> w548
                      tunnel: [w550 w562] -> w547
                      tunnel: w544 -> [w554 w566]
                      frame False {
                        w556 = "'" ("String")
                        # "Abfrage ob zwischen 2-5 Uhr? (nein)\nLaden vom öfftl. Netz"
                        n200 = property on="Control-Matrix-Overview" class="MehrSpaltFeld (strikt)"() -> ("ColHdrString"=w549:string[])  [unwired: 2 in, 2 out]
                        n201 = Unbundle By Name(w553) -> ("DataHandling"=w561:refnum<class "DataHandler.lvclass">)
                        n202 = Concatenate Strings(w556, "0" ("String"), w556) -> (w558:string)
                        n203 = Index Array(array=w549, index=5) -> (element=w560:string)
                        n204 = call-dynamic "setValueDH.vi"("TableName"=w554, "error in (no error)"=w552, "Value"=w558, "ItemName"=w560, "DataHandler in"=w561) -> ("error out"=w551:errorcluster, "DataHandler out"=w559:refnum<class "DataHandler.lvclass">)  [unwired: 5 in]
                        n205 = Bundle By Name(cluster=w553, "DataHandling"=w559) -> (w550:T2)
                      }
                      frame True {
                        w568 = "'" ("String")
                        # "Abfrage ob zwischen 2-5 Uhr? (ja)\nLaden vom öfftl. Netz"
                        n206 = property on="Control-Matrix-Overview" class="MehrSpaltFeld (strikt)"() -> ("ColHdrString"=w570:string[])  [unwired: 2 in, 2 out]
                        n207 = Unbundle By Name(w565) -> ("DataHandling"=w574:refnum<class "DataHandler.lvclass">)
                        n208 = Concatenate Strings(w568, "1.375" ("String"), w568) -> (w571:string)
                        n209 = Index Array(array=w570, index=5) -> (element=w573:string)
                        n210 = call-dynamic "setValueDH.vi"("TableName"=w566, "error in (no error)"=w564, "Value"=w571, "ItemName"=w573, "DataHandler in"=w574) -> ("error out"=w563:errorcluster, "DataHandler out"=w572:refnum<class "DataHandler.lvclass">)  [unwired: 5 in]
                        n211 = Bundle By Name(cluster=w565, "DataHandling"=w572) -> (w562:T2)
                      }
                    }
                  }
                }
              }
            }
            n212 = Bundle By Name(cluster=w425, "Zone 3"=w426) -> (w424:T3)
          }
        }
        "Load Limit" <- w117
        "Unload Limit" <- w116
      }
      event "Stopp": Value Change {
        w582 = "'" ("String")
        # "Load Power Limit"
        n213 = event-data() -> ()  [unwired: 1 in, 6 out]
        n214 = property on="Control-Matrix-Overview" class="MehrSpaltFeld (strikt)"() -> ("ColHdrString"=w580:string[])  [unwired: 2 in, 2 out]
        n215 = Unbundle By Name(w577) -> ("DataHandler out"=w583:refnum<class "DataHandler.lvclass">)
        n216 = Concatenate Strings(w582, "1" ("String"), w582) -> (w585:string)
        n217 = Index Array(array=w580, index=1) -> (element=w586:string)
        n218 = call-dynamic "setValueDH.vi"("TableName"=w575, "error in (no error)"=w579, "Value"=w585, "ItemName"=w586, "DataHandler in"=w583) -> ("error out"=w578:errorcluster, "DataHandler out"=w584:refnum<class "DataHandler.lvclass">)  [unwired: 5 in]
        n219 = Bundle By Name(cluster=w577, "DataHandler out"=w584) -> (w576:T5)
      }
    }
    "error out 2" <- w67
    n220 = Bundle By Name(cluster=w67, "status"=w70) -> (w69:errorcluster)
    n221 = Or(x=w67, y=w69) -> (x .or. y?=w68:bool)
  }
  n222 = case shown="True" w11 {
    tunnel: w12 -> [w590 w593]
    tunnel: w8 -> [w589 w592]
    tunnel: [w589 w591] -> w7
    frame False {
      "DataFlowOUT" <- w590
    }
    frame True {
      n223 = Unbundle By Name(w593) -> ("DataCollector out"=w595:refnum<class "DataCollector.lvclass">, "DataHandler out"=w594:refnum<class "DataHandler.lvclass">)
      n224 = call "CloseCollector.vi"("error in (no error)"=w592, "DataCollector in"=w595) -> ("error out"=w596:errorcluster)  [unwired: 8 in, 1 out]
      n225 = call-dynamic "CloseHandler.vi"("error in (no error)"=w596, "DataHandling in"=w594) -> ("error out"=w591:errorcluster)  [unwired: 8 in, 1 out]
    }
  }
  "error out" <- w7
